vi "SLM Mask Select 640.vi"(4 "error in (no error)":errorcluster, 5 "ACTIVE MASK":u16(ring) items=[" MASTER", " SLAVE"], 7 "VISA Resource Name":refnum<visa-resource-name>) -> (0 "error out":errorcluster)   [LabVIEW 2022 SP3]
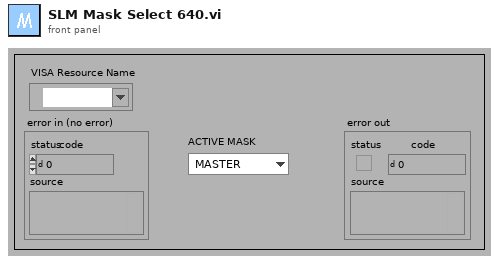
[diagram p1: front panel]
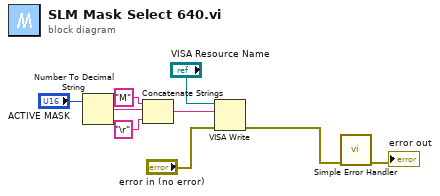
[diagram p0: block diagram]
diagram:
  n1 = Number To Decimal String(number="ACTIVE MASK") -> (decimal integer string=w5:string)  [unwired: 1 in]
  n2 = Concatenate Strings("M" ("Substring"), w5, "\r" ("Substring")) -> (w3:string)
  n3 = VISA Write(VISA resource name="VISA Resource Name", write buffer=w3, error in (no error)="error in (no error)") -> (error out=w1:errorcluster)  [unwired: 2 out]
  n4 = call <vilib>:"Simple Error Handler.vi"("error in (no error)"=w1) -> ("error out"=→"error out":errorcluster)  [unwired: 4 in, 4 out]
